vi "Acquire.vi"() -> ()   [LabVIEW 2015]
uses:
  <vilib>/vision/NI_Vision_Development_Module.lvlib
panel:
  in  "Delay (s.)":dbl(slide)=0.995260663507109 scale=0.0..3.0
  out "Pass Status":bool
  in  "Max Distance":dbl=4.0 min=0.0 format="%.2f"
  out "Distance":dbl[](graph) caption="Distance of Contour from Fitted Circle"
  out "Image 4":T1(plugin-control)
  out "BarCode Found?":bool
  out "Barcode Read":cluster{"Data":string, "Barcode Type":string}[](array[cluster])
  out "Number of Barcodes Found":u32
  out "Image":T1(plugin-control)
  out "Image 3":T1(plugin-control)
  out "Image 2":T1(plugin-control)
  out "x > y?":bool
  out "Mean Value":sgl
  in  "stop":bool
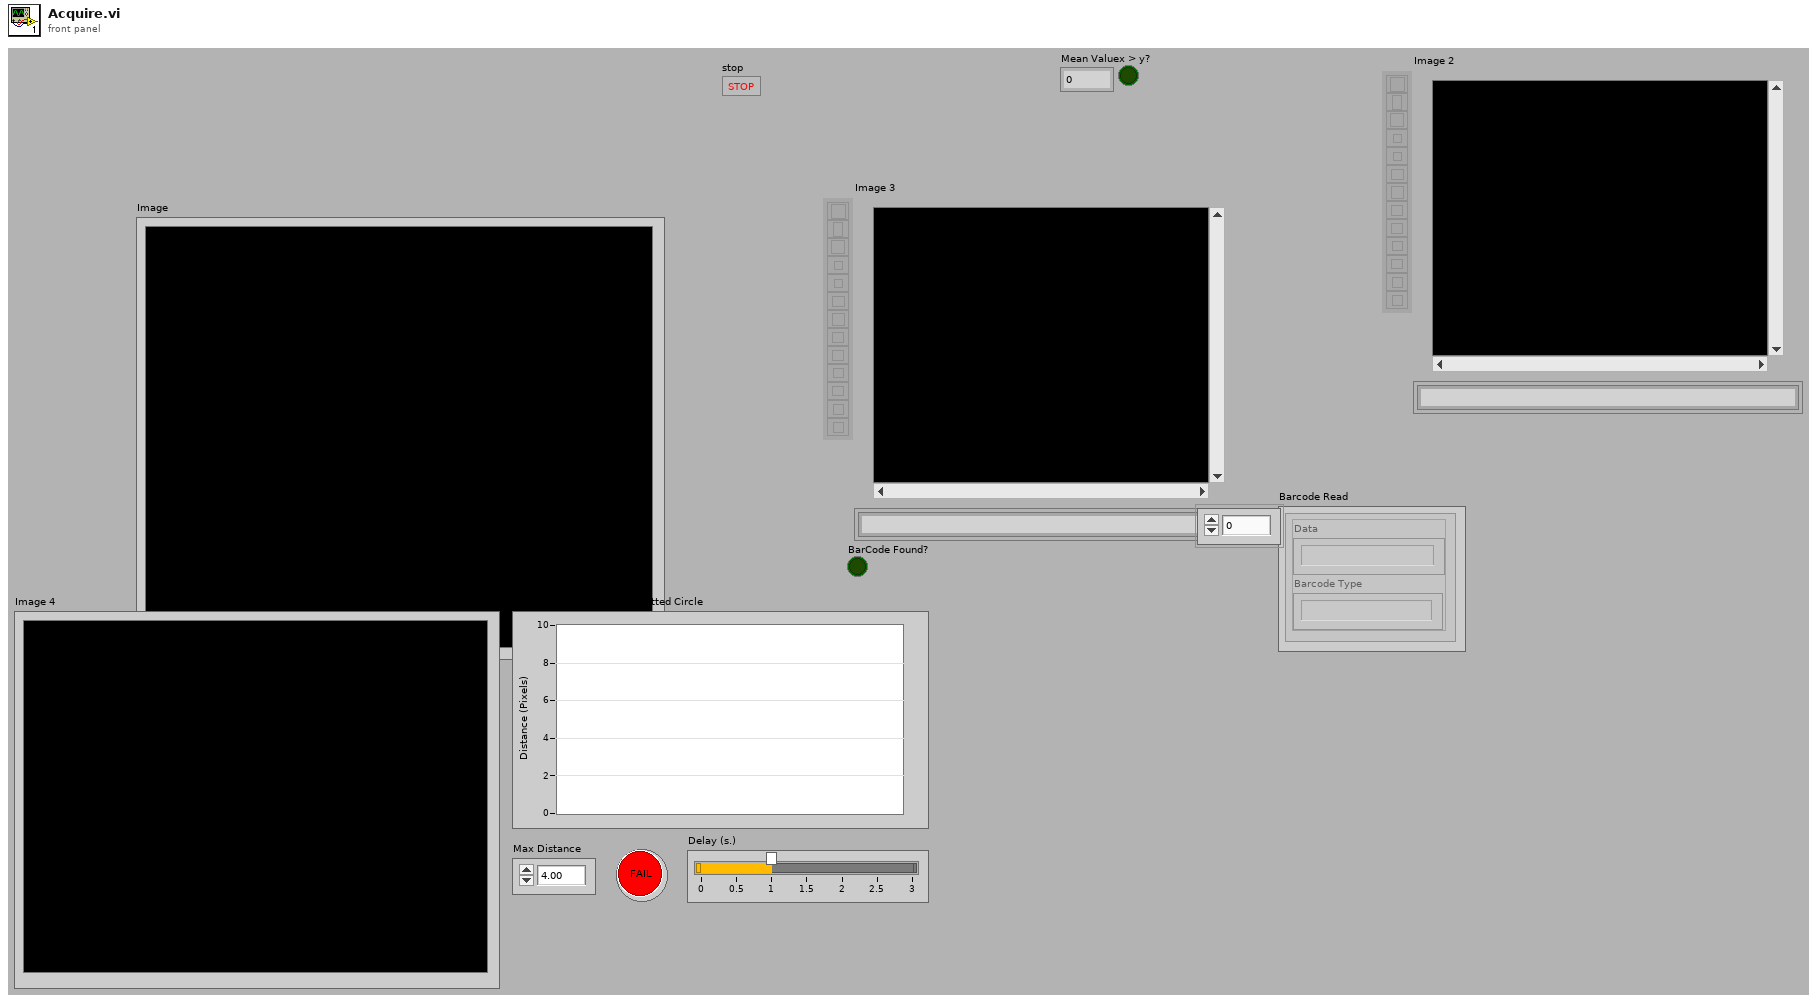
[diagram p1: front panel]
types:
  T1 = typedef "IMAQ Image.ctl" = refnum<image>
  T2 = typedef "IMAQ Rectangle" = cluster{"Left":i32, "Top":i32, "Right":i32, "Bottom":i32, "Rotation":dbl}
  T3 = typedef "ROI Descriptor" = cluster{"Global Rectangle":i32[], "Contours":cluster{"ID":enum32{"External", "Internal"}, "Type":u32, "Coordinates":i32[]}[]}
  T4 = typedef "IMAQ Circle" = cluster{"Center X":i32, "Center Y":i32, "Inner Radius":i32, "Outer Radius":i32, "Start Angle":dbl, "End Angle":dbl}
  T5 = cluster{"Overlay?":bool, "Color":u32, "Width":u32, "Maintain Width?":bool}
  T6 = enum16{"Closest To Search Start", "Maximum Length", "Strongest Mean Gradient Change"}
  T7 = enum16{"Rect Left To Right", "Rect Right To Left", "Rect Top To Bottom", "Rect Bottom To Top", "Annulus Inner To Outer", "Annulus Outer To Inner", "Annulus Start Angle To End Angle", "Annulus End Angle To Start Angle"}
  T8 = cluster{"Target Point":cluster{"X":dbl, "Y":dbl}, "Template Point":cluster{"X":dbl, "Y":dbl}, "Distance":dbl}[]
  T9 = cluster{"Mean Value":sgl, "Standard Variation":sgl, "Minimal Value":sgl, "Maximal Value":sgl, "Area (calibrated)":sgl, "Area (pixels)":i32, "%":sgl}
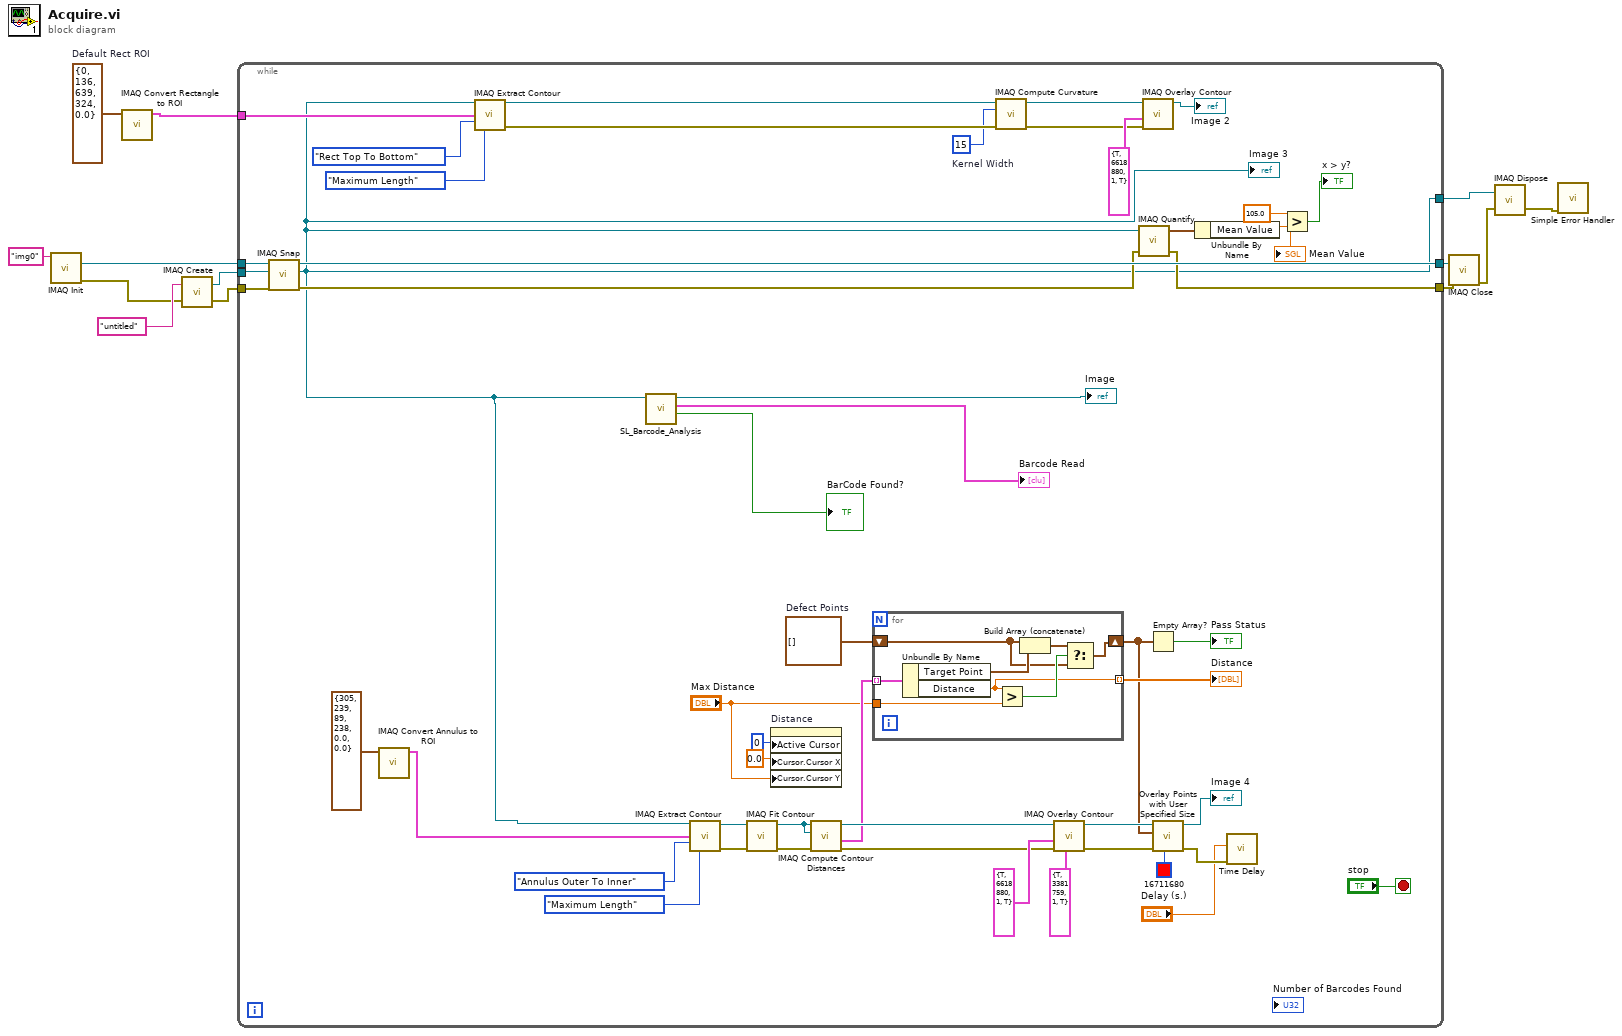
[diagram p0: block diagram]
diagram:
  w2 = T2 {"Left"=0, "Top"=136, "Right"=639, "Bottom"=324, "Rotation"=0.0}  # Default Rect ROI
  n1 = call <vilib>:"IMAQ Init.vi"("Interface Name"="img0") -> ("error out"=w6:errorcluster, "IMAQ Session Out"=w7:refnum<k11>)  [unwired: 9 in]
  n2 = call "IMAQ Convert Rectangle to ROI"("Rectangle"=w2) -> ("ROI Descriptor"=w1:T3)  [unwired: 8 in, 1 out]
  n3 = call "IMAQ Create"("Image Name"="untitled", "error in (no error)"=w6) -> ("New Image"=w11:T1, "error out"=w12:errorcluster)  [unwired: 3 in]
  n4 = while {
    tunnel: w12 -> [w63]
    tunnel: w11 -> [w62]
    tunnel: w7 -> [w61]
    tunnel: [w58] -> w5
    tunnel: [w60] -> w4
    tunnel: [w16] -> w3
    tunnel: w1 -> [w44]
    stop <- "stop" stop-if-true
    w27 = cluster{"X":dbl, "Y":dbl}[] []  # Defect Points
    w47 = u32 15  # Kernel Width
    n5 = call <vilib>:"IMAQ Snap.vi"("error in (no error)"=w63, "Image In"=w62, "IMAQ Session In"=w61) -> ("error out"=w59:errorcluster, "Image Out"=w16:T1, "IMAQ Session Out"=w60:refnum<k11>)  [unwired: 6 in]
    "Image 3" <- w16
    n6 = call "IMAQ Convert Annulus to ROI"("Annulus"=T4 {"Center X"=305, "Center Y"=239, "Inner Radius"=89, "Outer Radius"=238, "Start Angle"=0.0, "End Angle"=0.0}) -> ("ROI Descriptor"=w14:T3)  [unwired: 8 in, 1 out]
    n7 = call "IMAQ Extract Contour"("Source Image"=w16, "ROI Descriptor"=w44, "Search Direction"=T7."Rect Top To Bottom", "Contour Selection"=T6."Maximum Length") -> ("Source Image Out"=w46:T1, "error out"=w50:errorcluster)  [unwired: 4 in, 6 out]
    n8 = call "SL_Barcode_Analysis.vi"("Refnum in"=w16) -> ("BarCode Found?"=→"BarCode Found?":bool, "Barcode Read"=→"Barcode Read":cluster{"Data":string, "Barcode Type":string}[], "Refnum out"=→"Image":T1)  [unwired: 8 in]
    n9 = call "IMAQ Extract Contour"("Source Image"=w16, "ROI Descriptor"=w14, "Search Direction"=T7."Annulus Outer To Inner", "Contour Selection"=T6."Maximum Length") -> ("Source Image Out"=w33:T1, "error out"=w32:errorcluster)  [unwired: 4 in, 6 out]
    n10 = call-poly "IMAQ Fit Contour"("error in (no error)"=w32, "Contour Image"=w33) -> ("error out"=w38:errorcluster, "Contour Image Out"=w29:T1)  [unwired: 2 in, 6 out]
    n11 = property on="Distance" class="WFGraph (strict)"("Active Cursor"=u32 0, "Cursor.Cursor X"=0.0 ("Cursor.Cursor Position:Cursor X"), "Cursor.Cursor Y"="Max Distance") -> ()  [unwired: 2 in, 2 out]
    n12 = call "IMAQ Compute Contour Distances"("error in (no error)"=w38, "Template Contour Image"=w29, "Target Contour Image"=w29) -> ("error out"=w34:errorcluster, "Distances"=w28:T8, "Target Contour Image Out (dup)"=w35:T1)  [unwired: 2 in, 4 out]
    n13 = for {
      tunnel: w28 -> [w72] mode=indexing
      shift-right: [w67] -> w22
      shift-left: w27 -> [w68]
      tunnel: [w66] -> w23 mode=indexing
      tunnel: "Max Distance" -> [w65]
      n14 = Unbundle By Name(w72) -> ("Target Point"=w71:cluster{"X":dbl, "Y":dbl}, "Distance"=w66:dbl)
      n15 = Greater?(x=w66, y=w65) -> (0:w70:bool)
      n16 = Build Array (concatenate)(w68, w71) -> (w69:cluster{"X":dbl, "Y":dbl}[])
      n17 = Select(t=w69, s=w70, f=w68) -> (s? t:f=w67:cluster{"X":dbl, "Y":dbl}[])
    }
    "Distance" <- w23
    n18 = call "IMAQ Compute Curvature"("error in (no error)"=w50, "Kernel Width"=w47, "Contour Image"=w46) -> ("error out"=w49:errorcluster, "Contour Image Out (dup)"=w48:T1)  [unwired: 7 out]
    n19 = call "IMAQ Overlay Contour"("Contour Equation Settings"=T5 {"Overlay?"=TRUE, "Color"=3381759, "Width"=1, "Maintain Width?"=TRUE}, "error in (no error)"=w34, "Contour Points Settings"=T5 {"Overlay?"=TRUE, "Color"=6618880, "Width"=1, "Maintain Width?"=TRUE}, "Image"=w35) -> ("error out"=w17:errorcluster, "Image Out"=w26:T1)  [unwired: 2 in, 4 out]
    n20 = call "IMAQ Quantify"("error in (no error)"=w59, "Image"=w16) -> ("error out"=w58:errorcluster, "Global Report"=w57:T9)  [unwired: 1 in, 1 out]
    n21 = call "IMAQ Overlay Contour"("error in (no error)"=w49, "Contour Points Settings"=T5 {"Overlay?"=TRUE, "Color"=6618880, "Width"=1, "Maintain Width?"=TRUE}, "Image"=w48) -> ("Image Out"=→"Image 2":T1)  [unwired: 3 in, 5 out]
    n22 = Empty Array?(array=w22) -> (empty?=→"Pass Status":bool)
    n23 = call "Overlay Points with User Specified Size.vi"("Color"=u32 16711680, "error in"=w17, "Points"=w22, "Image In"=w26) -> ("error out"=w19:errorcluster, "Image Out"=→"Image 4":T1)  [unwired: 6 in]
    n24 = Unbundle By Name(w57) -> ("Mean Value"=w56:sgl)
    "Mean Value" <- w56
    n25 = call "Time Delay"("error in (no error)"=w19, "Delay Time (s)"="Delay (s.)") -> ()  [unwired: 9 in, 1 out]
    n26 = Greater?(x=sgl 105.0, y=w56) -> (0:→"x > y?":bool)
  }
  n27 = call <vilib>:"IMAQ Close.vi"("error in (no error)"=w5, "IMAQ Session In"=w4) -> ("error out"=w10:errorcluster)  [unwired: 9 in]
  n28 = call "IMAQ Dispose"("Image"=w3, "error in (no error)"=w10) -> ("error out"=w8:errorcluster)  [unwired: 4 in]
  n29 = call <vilib>:"Simple Error Handler.vi"("error in (no error)"=w8) -> ()  [unwired: 4 in, 5 out]
